vi "题目5.vi"() -> ()   [LabVIEW 2017]
panel:
  out "恭喜":bool
  out "通过":bool
  out "警告":bool
  in  "x":dbl
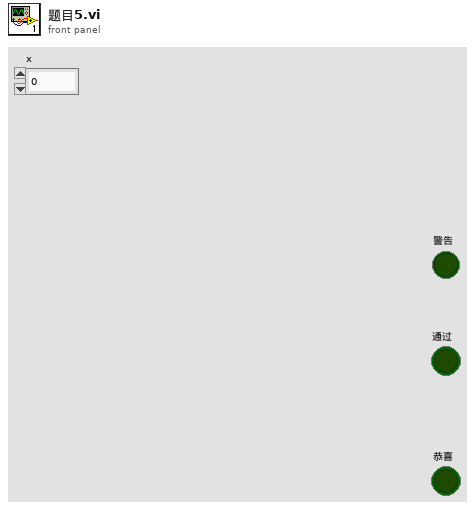
[diagram p1: front panel]
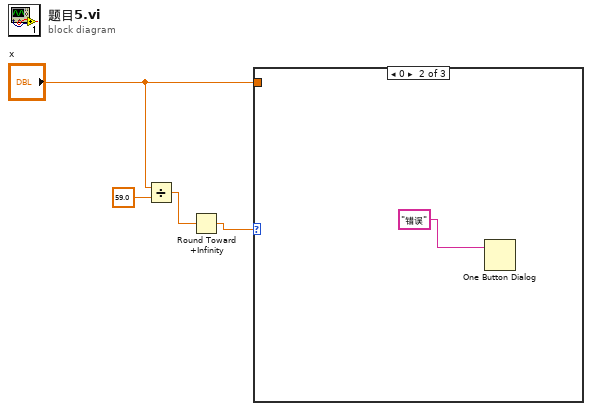
[diagram p0: block diagram]
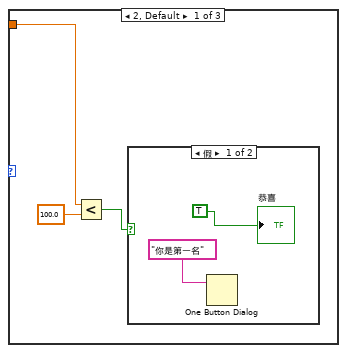
[diagram p2: hidden frame]
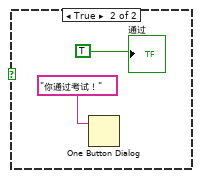
[diagram p3: hidden frame]
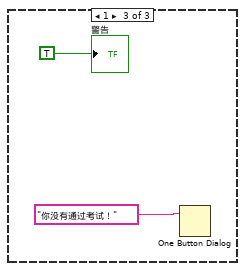
[diagram p4: hidden frame]
diagram:
  n1 = Divide(x="x", y=59.0) -> (x/y=w3:dbl)
  n2 = Round Toward +Infinity(x=w3) -> (ceil(x): smallest int >= x=w2:dbl)
  n3 = case shown="0" w2 {
    tunnel: "x" -> [w7 _ _]
    frame 2, Default {
      n4 = Less?(x=w7, y=100.0) -> (x < y?=w5:bool)
      n5 = case shown="假" w5 {
        frame False {
          n6 = One Button Dialog(message="你是第一名") -> ()  [unwired: 1 in, 1 out]
          "恭喜" <- TRUE
        }
        frame True {
          n7 = One Button Dialog(message="你通过考试！") -> ()  [unwired: 1 in, 1 out]
          "通过" <- TRUE
        }
      }
    }
    frame 0 {
      n8 = One Button Dialog(message="错误") -> ()  [unwired: 1 in, 1 out]
    }
    frame 1 {
      n9 = One Button Dialog(message="你没有通过考试！") -> ()  [unwired: 1 in, 1 out]
      "警告" <- TRUE
    }
  }
